vi "COM_1.vi"() -> ()   [LabVIEW 2011]
uses:
  <vilib>/Instr/_visa.llb/VISA Configure Serial Port (Instr).vi
panel:
  out "值":cluster{enum16{"tt", "wwww"}, string[]}
  out "连接的字符串":string
  out "错误输出":errorcluster
  out "读取缓冲区":string
  out "返回数":u32
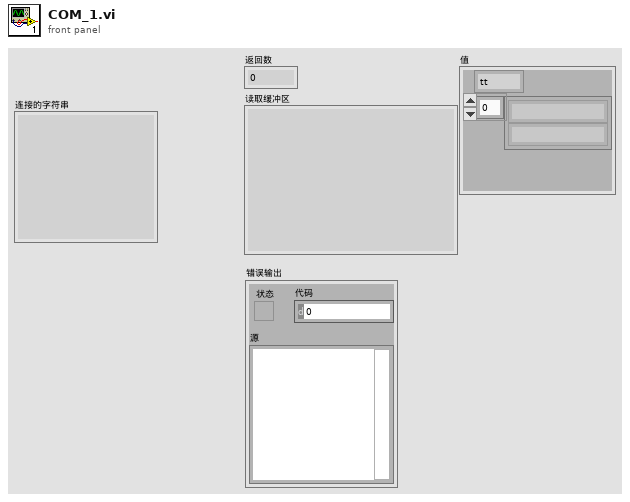
[diagram p1: front panel]
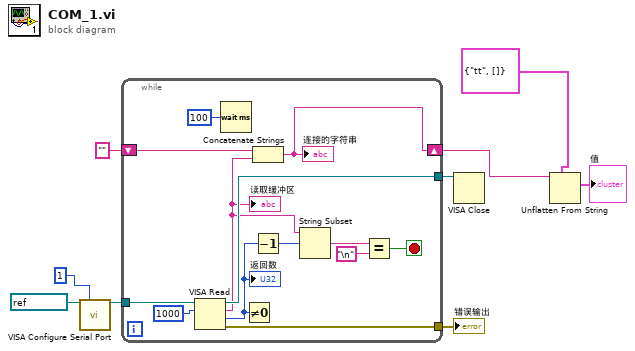
[diagram p0: block diagram]
diagram:
  n1 = call-poly "VISA Configure Serial Port"("VISA resource name"=refnum<visa-resource-name> "COM3", "timeout (10sec)"=u32 1) -> ("VISA resource name out"=w8:refnum<visa-resource-name>)  [unwired: 12 in, 1 out]
  n2 = while {
    tunnel: w8 -> [w21]
    tunnel: [w20] -> w7
    tunnel: [w19] -> w5
    shift-right: [w17] -> w3
    shift-left: "" ("read buffer") -> [w18]
    stop <- w11 stop-if-true
    n3 = VISA Read(VISA resource name=w21, byte count=u32 1000 ("字节总数")) -> (VISA resource name out=w19:refnum<visa-resource-name>, read buffer=w16:string, return count=w15:u32, error out=w20:errorcluster)  [unwired: 1 in]
    "返回数" <- w15
    "读取缓冲区" <- w16
    n4 = Wait (ms)(milliseconds to wait=u32 100 ("等待时间（毫秒）")) -> ()  [unwired: 1 out]
    n5 = Not Equal To 0?(x=w15) -> ()  [unwired: 1 out]
    n6 = Concatenate Strings(w18, w16) -> (w17:string)
    "连接的字符串" <- w17
    n7 = Decrement(x=w15) -> (x-1=w14:u32)
    n8 = String Subset(string=w16, offset (0)=w14) -> (substring=w13:string)  [unwired: 1 in]
    n9 = Equal?(x=w13, y="\n") -> (x = y?=w11:bool)
  }
  "错误输出" <- w7
  n10 = VISA Close(VISA resource name=w5) -> ()  [unwired: 1 in, 1 out]
  n11 = Unflatten From String(type=cluster{enum16{"tt", "wwww"}, string[]} {enum."tt", []}, binary string=w3) -> (value=→"值":cluster{enum16{"tt", "wwww"}, string[]})  [unwired: 3 in, 2 out]
